vi "MccHat_Global.vi"() -> ()   [LabVIEW 2019]
panel:
  out "chart_temp":waveform(dbl)[](graph)=[{"t0"=timestamp(3772890114.31303 s since 1904-01-01), "dt"=1.0, "Y"=[0.8687935985565186]}, {"t0"=timestamp(3772890114.31303 s since 1904-01-01), "dt"=1.0, "Y"=[86.87935985565186]}, {"t0"=timestamp(3772890114.31303 s since 1904-01-01), "dt"=1.0, "Y"=[30.48853325313992]}, {"t0"=timestamp(3772890114.31303 s since 1904-01-01), "dt"=1.0, "Y"=[303.6385332531399]}]
  out "MccHat_ST":u32(colorbox)
  out "MccHat_P":dbl format="%.1f"
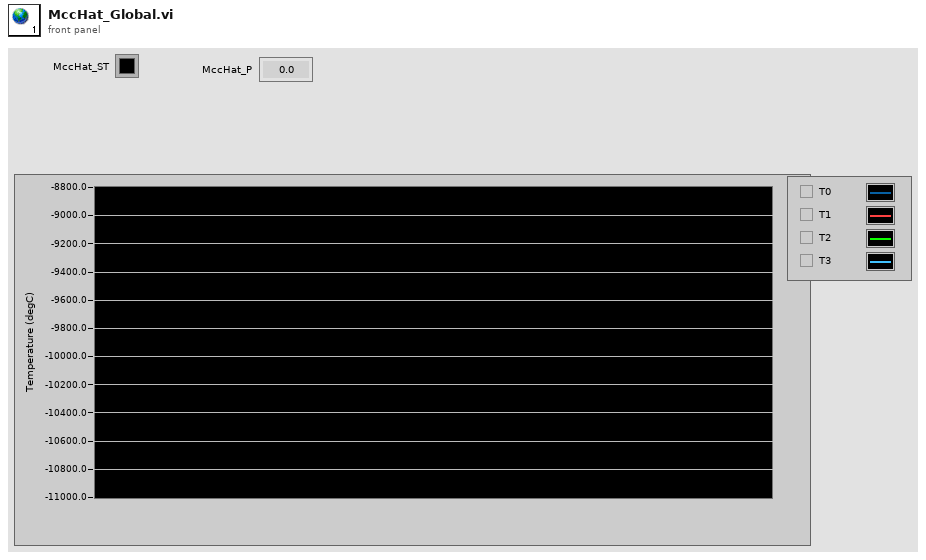
[diagram p1: front panel]
diagram:
